vi "FGV_PSP - VRM Targets.vi"(4 "error in":errorcluster, 6 "Function":enum16{"write", "read"}(ring), 7 "VRM Targets":T1) -> (0 "error out":errorcluster, 3 "VRM Targets 2":T1)   [LabVIEW 2016]
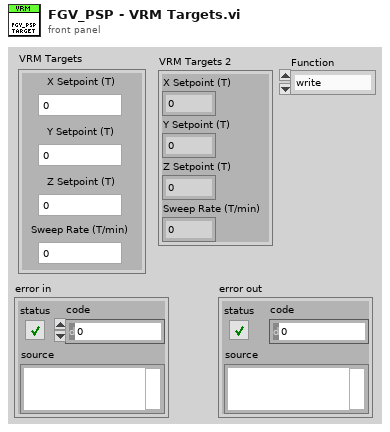
[diagram p1: front panel]
types:
  T1 = cluster{"X Setpoint (T)":dbl, "Y Setpoint (T)":dbl, "Z Setpoint (T)":dbl, "Sweep Rate (T/min)":dbl}
  T2 = cluster{"[0]":dbl, "[1]":dbl, "[2]":dbl, "[3]":dbl}
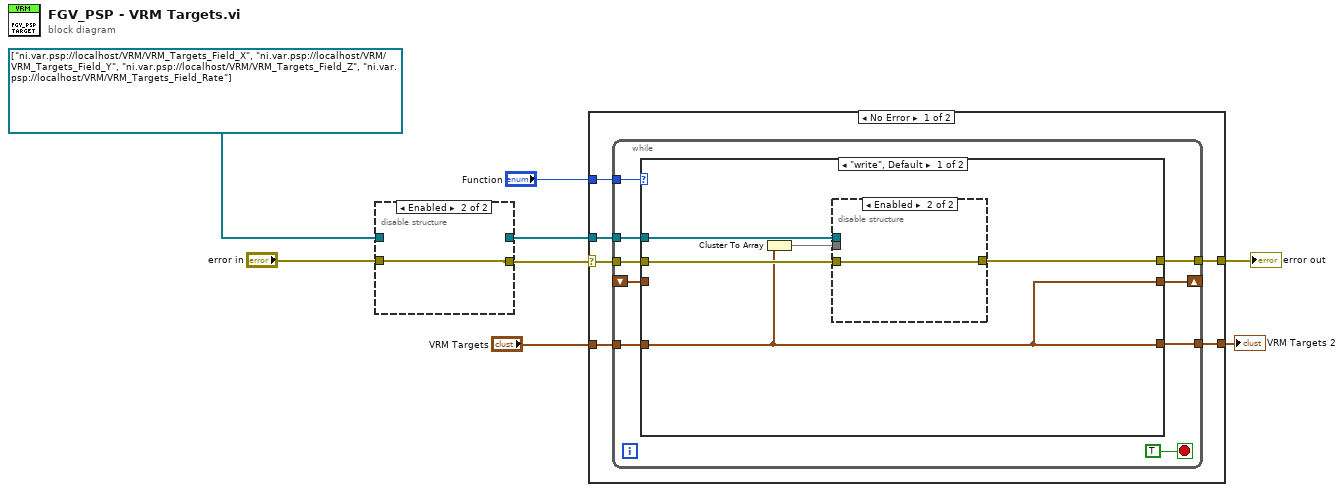
[diagram p0: block diagram]
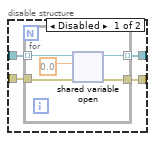
[diagram p2: hidden frame]
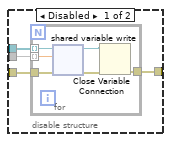
[diagram p3: hidden frame]
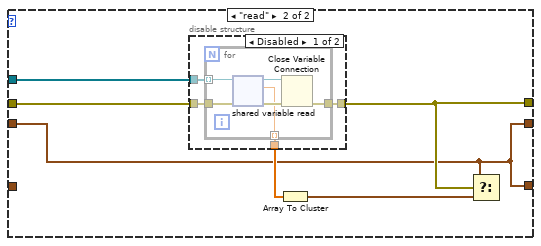
[diagram p4: hidden frame]
diagram:
  n1 = disable-structure shown="Enabled" {
    disable-tunnel: [w12 _] -> w6
    disable-tunnel: [w11 w18] -> w5
    disable-tunnel: "error in" -> [w10 w18]
    disable-tunnel: refnum<k21>[] ["ni.var.psp://localhost/VRM/VRM_Targets_Field_X", "ni.var.psp://localhost/VRM/VRM_Targets_Field_Y", "ni.var.psp://localhost/VRM/VRM_Targets_Field_Z", "ni.var.psp://localhost/VRM/VRM_Targets_Field_Rate"] -> [w9 _]
    frame Disabled {
      n2 = for {
        tunnel: [w17] -> w12 mode=indexing
        tunnel: [w16] -> w11
        tunnel: w10 -> [w15]
        tunnel: w9 -> [w14] mode=indexing
        n3 = shared-variable-open(w14, w15, 0.0) -> (w17:refnum<k21>, w16:errorcluster)  [unwired: 1 in]
      }
    }
    frame Enabled {
    }
  }
  n4 = case shown="No Error" w5 {
    selector: w5 -> [w24 w67]
    tunnel: [w23 w67] -> w8
    tunnel: [w22 w66] -> w3
    tunnel: "Function" -> [w21 _]
    tunnel: w6 -> [w20 _]
    tunnel: "VRM Targets" -> [w19 w66]
    frame No Error {
      n5 = while {
        shift-right: [w28] -> _
        shift-left: _ -> [w27]
        tunnel: w24 -> [w32]
        tunnel: [w31] -> w23
        tunnel: [w30] -> w22
        tunnel: w21 -> [w29]
        tunnel: w20 -> [w26]
        tunnel: w19 -> [w25]
        stop <- TRUE stop-if-true
        n6 = case shown="\"write\", Default" w29 {
          tunnel: w32 -> [w37 w54]
          tunnel: [w38 w53] -> w31
          tunnel: [w34 w50] -> w30
          tunnel: [w34 w50] -> w28
          tunnel: w27 -> [_ w50]
          tunnel: w26 -> [w36 w55]
          tunnel: w25 -> [w34 _]
          frame "write", Default {
            n7 = Cluster To Array(cluster=w34) -> (array=w35:dbl[])
            n8 = disable-structure shown="Enabled" {
              disable-tunnel: [w42 w49] -> w38
              disable-tunnel: w37 -> [w41 w49]
              disable-tunnel: w36 -> [w40 _]
              disable-tunnel: w35 -> [w39 _]
              frame Disabled {
                n9 = for {
                  tunnel: [w47] -> w42
                  tunnel: w41 -> [w45]
                  tunnel: w40 -> [w44] mode=indexing
                  tunnel: w39 -> [w43] mode=indexing
                  n10 = shared-variable-write(w44, w45, w43) -> (w46:refnum<k21>, w48:errorcluster)
                  n11 = Close Variable Connection(8:w48, 11:w46) -> (0:w47:errorcluster)
                }
              }
              frame Enabled {
              }
            }
          }
          frame "read" {
            n12 = disable-structure shown="Disabled" {
              disable-tunnel: w55 -> [w59 _]
              disable-tunnel: w54 -> [w58 _]
              disable-tunnel: [w57 _] -> w53
              disable-tunnel: [w56 _] -> w52
              frame Disabled {
                n13 = for {
                  tunnel: [w63] -> w57
                  tunnel: w59 -> [w62] mode=indexing
                  tunnel: w58 -> [w61]
                  tunnel: [w60] -> w56 mode=indexing
                  n14 = shared-variable-read(w62, w61) -> (w65:refnum<k21>, w64:errorcluster, w60:dbl)  [unwired: 1 out]
                  n15 = Close Variable Connection(8:w64, 11:w65) -> (0:w63:errorcluster)
                }
              }
              frame Enabled {
              }
            }
            n16 = Array To Cluster(array=w52) -> (cluster=w51:T2)
            n17 = Select(t=w50, s=w53, f=w51) -> ()  [unwired: 1 out]
          }
        }
      }
    }
    frame Error {
    }
  }
  "error out" <- w8
  "VRM Targets 2" <- w3
